vi "Wavelength.vi"(4 "Fondo Scala AI1":dbl(ring)=5.0 items=["10"=10.0, "5"=5.0, "0.5"=0.5, "0.05"=0.05], 5 "Zero (Ch 1)":dbl=-0.085 format="%.3f", 6 "Zero (Ch 0)":dbl=0.013 format="%.3f", 8 "Fondo Scala AI0":dbl(ring)=5.0 items=["10"=10.0, "5"=5.0, "0.5"=0.5, "0.05"=0.05]) -> (0 "Lunghezza d'onda (nm)":dbl=nan format="%.3f", 1 "Rapporto":dbl=nan format="%.3f", 2 "V_1 (Volt)":dbl=-0.08488354506271055 format="%.3f", 3 "V_0 (Volt)":dbl=0.012553807393637543 format="%.3f")   [LabVIEW 2014]
doc: "Misuratore di lunghezza d'onda\nWS7.56-TO5"
uses:
  <vilib>/DAQmx/read.llb/DAQmx Read (Analog 2D DBL NChan NSamp).vi
  <vilib>/Analysis/baseanly.llb/Mean (DBL).vi
  <vilib>/DAQmx/create/channels.llb/DAQmx Create Channel (AI-Voltage-Basic).vi
  <vilib>/DAQmx/configure/timing.llb/DAQmx Timing (Sample Clock).vi
  <vilib>/DAQmx/miscellaneous.llb/DAQmx Fill In Error Info.vi
  <vilib>/Analysis/NI_AALBase.lvlib
panel:
  in  "physical channels 2":tag="Dev1/ai1"
  in  "physical channels":tag="Dev1/ai0"
  # "Collegare il  CB68 e CB33 alle due uscite. \nLa terra del circuito (CB29) DEVE essere in comune alla terra della scheda."
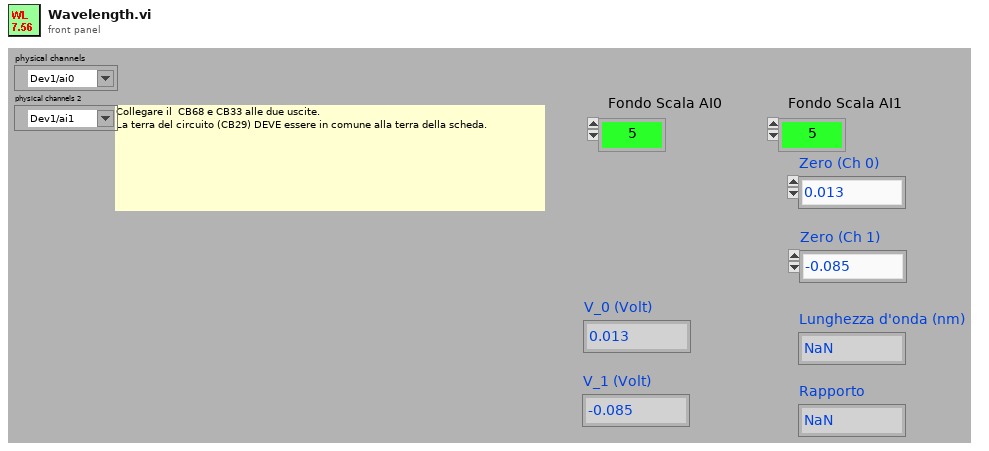
[diagram p1: front panel]
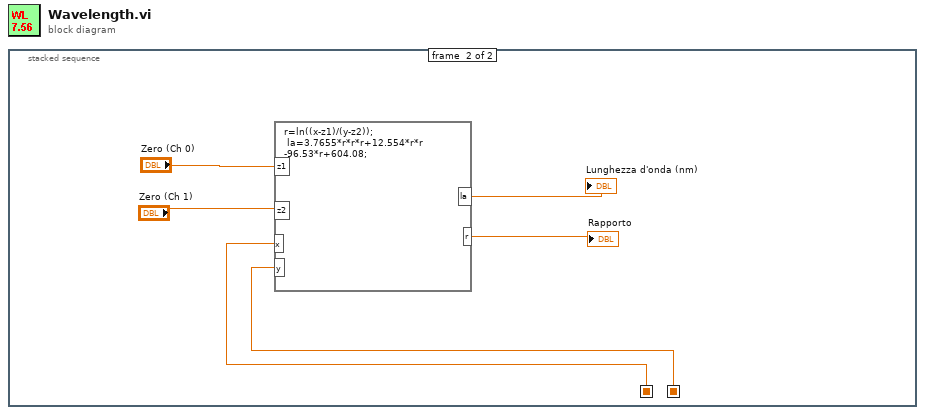
[diagram p0: block diagram]
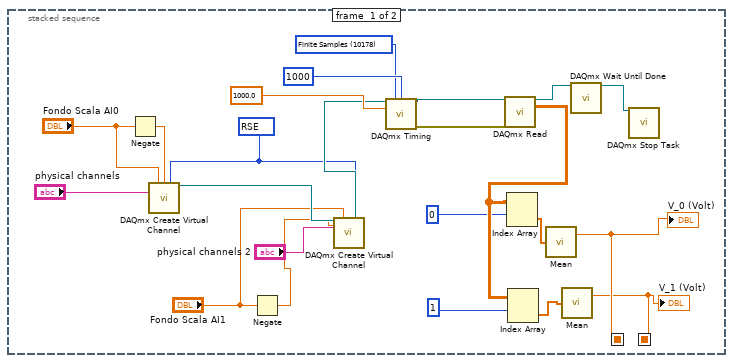
[diagram p2: hidden frame]
diagram:
  n1 = stacked-sequence {
    seq-local: [w9 _] -> [_ w27]
    seq-local: [w8 _] -> [_ w26]
    frame #0 {
      w16 = 10178 items=["Finite Samples"=10178, "Continuous Samples"=10123, "Hardware Timed Single Point"=12522] ("sample mode")
      w3 = 10083 items=["default"=-1, "RSE"=10083, "NRSE"=10078, "Differential"=10106, "Pseudodifferential"=12529] ("input terminal configuration")
      n2 = Negate(x="Fondo Scala AI0") -> (-x=w23:dbl)
      n3 = call-poly <vilib>:"DAQmx Create Virtual Channel.vi"("maximum value"="Fondo Scala AI0", "minimum value"=w23, "input terminal configuration"=w3, "physical channels"="physical channels") -> ("task out"=w7:refnum<k21>)  [unwired: 10 in, 1 out]
      n4 = Negate(x="Fondo Scala AI1") -> (-x=w5:dbl)
      n5 = call-poly <vilib>:"DAQmx Create Virtual Channel.vi"("task in"=w7, "maximum value"="Fondo Scala AI1", "minimum value"=w5, "input terminal configuration"=w3, "physical channels"="physical channels 2") -> ("task out"=w6:refnum<k21>)  [unwired: 9 in, 1 out]
      n6 = call-poly <vilib>:"DAQmx Timing.vi"("task/channels in"=w6, "sample mode"=w16, "samples per channel"=u32 1000, "rate"=1000.0) -> ("task out"=w21:refnum<k21>, "error out"=w20:errorcluster)  [unwired: 10 in]
      n7 = call-poly <vilib>:"DAQmx Read.vi"("task/channels in"=w21, "error in"=w20) -> ("task out"=w17:refnum<k21>, "data"=w14:dbl[][])  [unwired: 11 in, 1 out]
      n8 = Index Array(array=w14, index (row)=0) -> (element=w12:dbl[])  [unwired: 1 in]
      n9 = Index Array(array=w14, index (row)=1) -> (element=w11:dbl[])  [unwired: 1 in]
      n10 = call-poly <vilib>:"Mean.vi"("X"=w12) -> ("mean"=w9:dbl)  [unwired: 1 out]
      "V_0 (Volt)" <- w9
      n11 = call-poly <vilib>:"Mean.vi"("X"=w11) -> ("mean"=w8:dbl)  [unwired: 1 out]
      "V_1 (Volt)" <- w8
      n12 = call <vilib>:"DAQmx Wait Until Done.vi"("task/channels in"=w17) -> ("task out"=w15:refnum<k21>)  [unwired: 13 in, 1 out]
      n13 = call <vilib>:"DAQmx Stop Task.vi"("task/channels in"=w15) -> ()  [unwired: 13 in, 2 out]
    }
    frame #1 {
      n14 = formula code="r=ln((x-z1)/(y-z2));\n la=3.7655*r*r*r+12.554*r*r  -96.53*r+604.08;"("x"=w27, "y"=w26, "z1"="Zero (Ch 0)", "z2"="Zero (Ch 1)") -> ("la"=→"Lunghezza d'onda (nm)":dbl, "r"=→"Rapporto":dbl)
    }
  }
